vi "Sperre thrust alloc Neptune.vi"(0 "Thruster rpms":dbl[](array[numeric]), 1 "pan tilt":bool[](array[boolean]), 2 "Lights/HMI":bool[](array[boolean]), 5 "error in":errorcluster, 6 "dim 1":i8, 7 "Power Instruments":bool[](array[boolean]), 8 "dim 2":i8, 9 "Collecting Unit":bool[](array[boolean]), 10 "dim 34":i8, 11 "Zoom 1-2":bool[](array[boolean]), 12 "cam no":i8) -> (16 "telebuf out":u8[](array[numeric]), 19 "error IO":errorcluster)   [LabVIEW 2014]
uses:
  <vilib>/imath/engines/lvmath2/RunTimeEngine/BuiltInFunctions/uint8/NIMS_uint8(int).vi
  <instcachedir>/0/NIMS_uint8(int)_9D6EF81F86254677BB00410F9E5C6A1D.lvgen/NIMS_uint8(int)_9D6EF81F86254677BB00410F9E5C6A1D_001.vi
  <vilib>/imath/engines/lvmath2/RunTimeEngine/BuiltInFunctions/round/NIMS_round(DBL-S).vi
  <vilib>/imath/engines/lvmath2/RunTimeEngine/BuiltInFunctions/uint8/NIMS_uint8(real).vi
  <instcachedir>/0/NIMS_uint8(real)_CAA419FBB1354DA296C59E18C46DECF0.lvgen/NIMS_uint8(real)_CAA419FBB1354DA296C59E18C46DECF0_000.vi
  <instcachedir>/0/NIMS_uint8(int)_9D6EF81F86254677BB00410F9E5C6A1D.lvgen/NIMS_uint8(int)_9D6EF81F86254677BB00410F9E5C6A1D_000.vi
  <vilib>/imath/engines/lvmath2/RunTimeEngine/IndexReplace/NIMS V(S)=S.vi
  <instcachedir>/0/NIMS V(S)=S_2D52C4EC15D8415E870AEE69FB516CCA.lvgen/NIMS V(S)=S_2D52C4EC15D8415E870AEE69FB516CCA_003.vi
  <vilib>/imathl/engines/lvmath/Functions/Error Handling/Create Error.vi
  <vilib>/imath/engines/lvmath2/RunTimeEngine/BuiltInFunctions/bitand/NIMS_bitand(SorS,SorS).vi
  <instcachedir>/0/NIMS V(S)=S_2D52C4EC15D8415E870AEE69FB516CCA.lvgen/NIMS V(S)=S_2D52C4EC15D8415E870AEE69FB516CCA_000.vi
  <vilib>/imath/engines/lvmath2/RunTimeEngine/ErrorHandling/NIMS_Create Error From Enums.vi
  <vilib>/imath/engines/lvmath2/RunTimeEngine/IndexRead/NIMS V(S).vi
  <instcachedir>/0/NIMS V(S)_0488751826AF41519A22953C041130DC.lvgen/NIMS V(S)_0488751826AF41519A22953C041130DC_000.vi
  <vilib>/imath/engines/lvmath2/RunTimeEngine/BuiltInFunctions/bitset/NIMS_bitset(RS,RS,RS).vi
  <vilib>/imath/engines/lvmath2/RunTimeEngine/BuiltInFunctions/bitget/NIMS_bitget(SorS,SorS).vi
  <vilib>/imath/engines/lvmath2/RunTimeEngine/RangeToken/NIMS_Range_R2 - Integer.vi
  <instcachedir>/0/NIMS_Range_R2 - Integer_2D1304BAF97744E0A293025746CBADFC.lvgen/NIMS_Range_R2 - Integer_2D1304BAF97744E0A293025746CBADFC_000.vi
  <vilib>/imath/engines/lvmath2/RunTimeEngine/CommandStatement/MC_CommandStatement_break.vi
  <vilib>/imath/engines/lvmath2/RunTimeEngine/BuiltInFunctions/double/NIMS_double.vi
  <instcachedir>/0/NIMS_double_34E32F64C2B04A25A042F4CA881A0A41.lvgen/NIMS_double_34E32F64C2B04A25A042F4CA881A0A41_002.vi
  <vilib>/imath/engines/lvmath2/RunTimeEngine/BuiltInFunctions/mod/NIMS_mod_no_size_check.vi
  <instcachedir>/0/NIMS_mod_no_size_check_5393E3382FD241D281EEB71DA286C65B.lvgen/NIMS_mod_no_size_check_5393E3382FD241D281EEB71DA286C65B_001.vi
  <vilib>/imath/engines/lvmath2/RunTimeEngine/NodeEndStatement/NIMS_NodeEndStatement_Output.vi
  <instcachedir>/0/NIMS_NodeEndStatement_Output_53EC0D466D134D7ABD903AC30B43404B.lvgen/NIMS_NodeEndStatement_Output_53EC0D466D134D7ABD903AC30B43404B_011.vi
  <vilib>/imath/engines/lvmath2/RunTimeEngine/ErrorHandling/NIMS_Finalize Error.vi
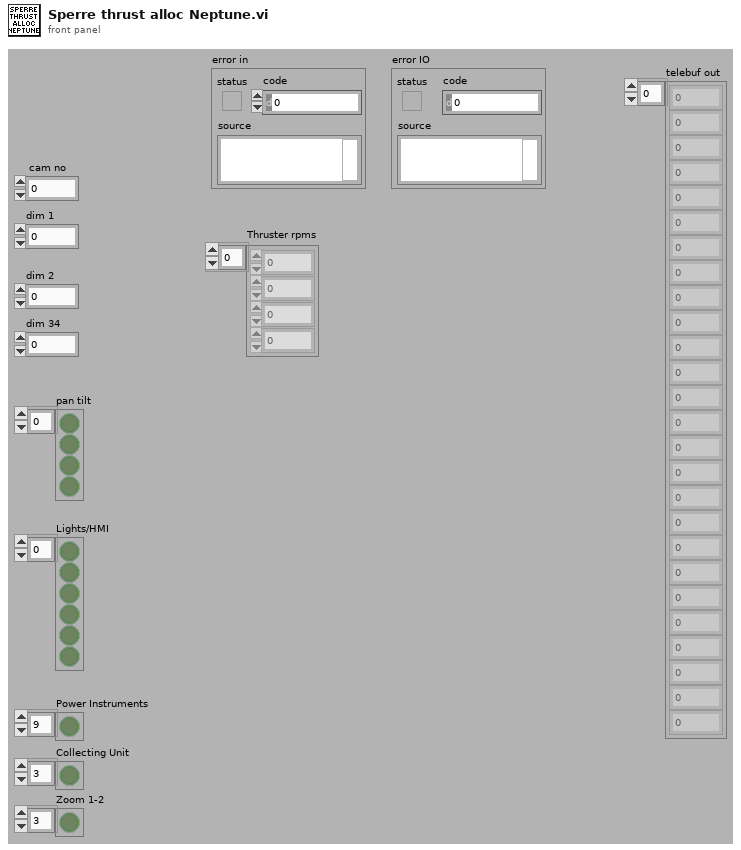
[diagram p1: front panel]
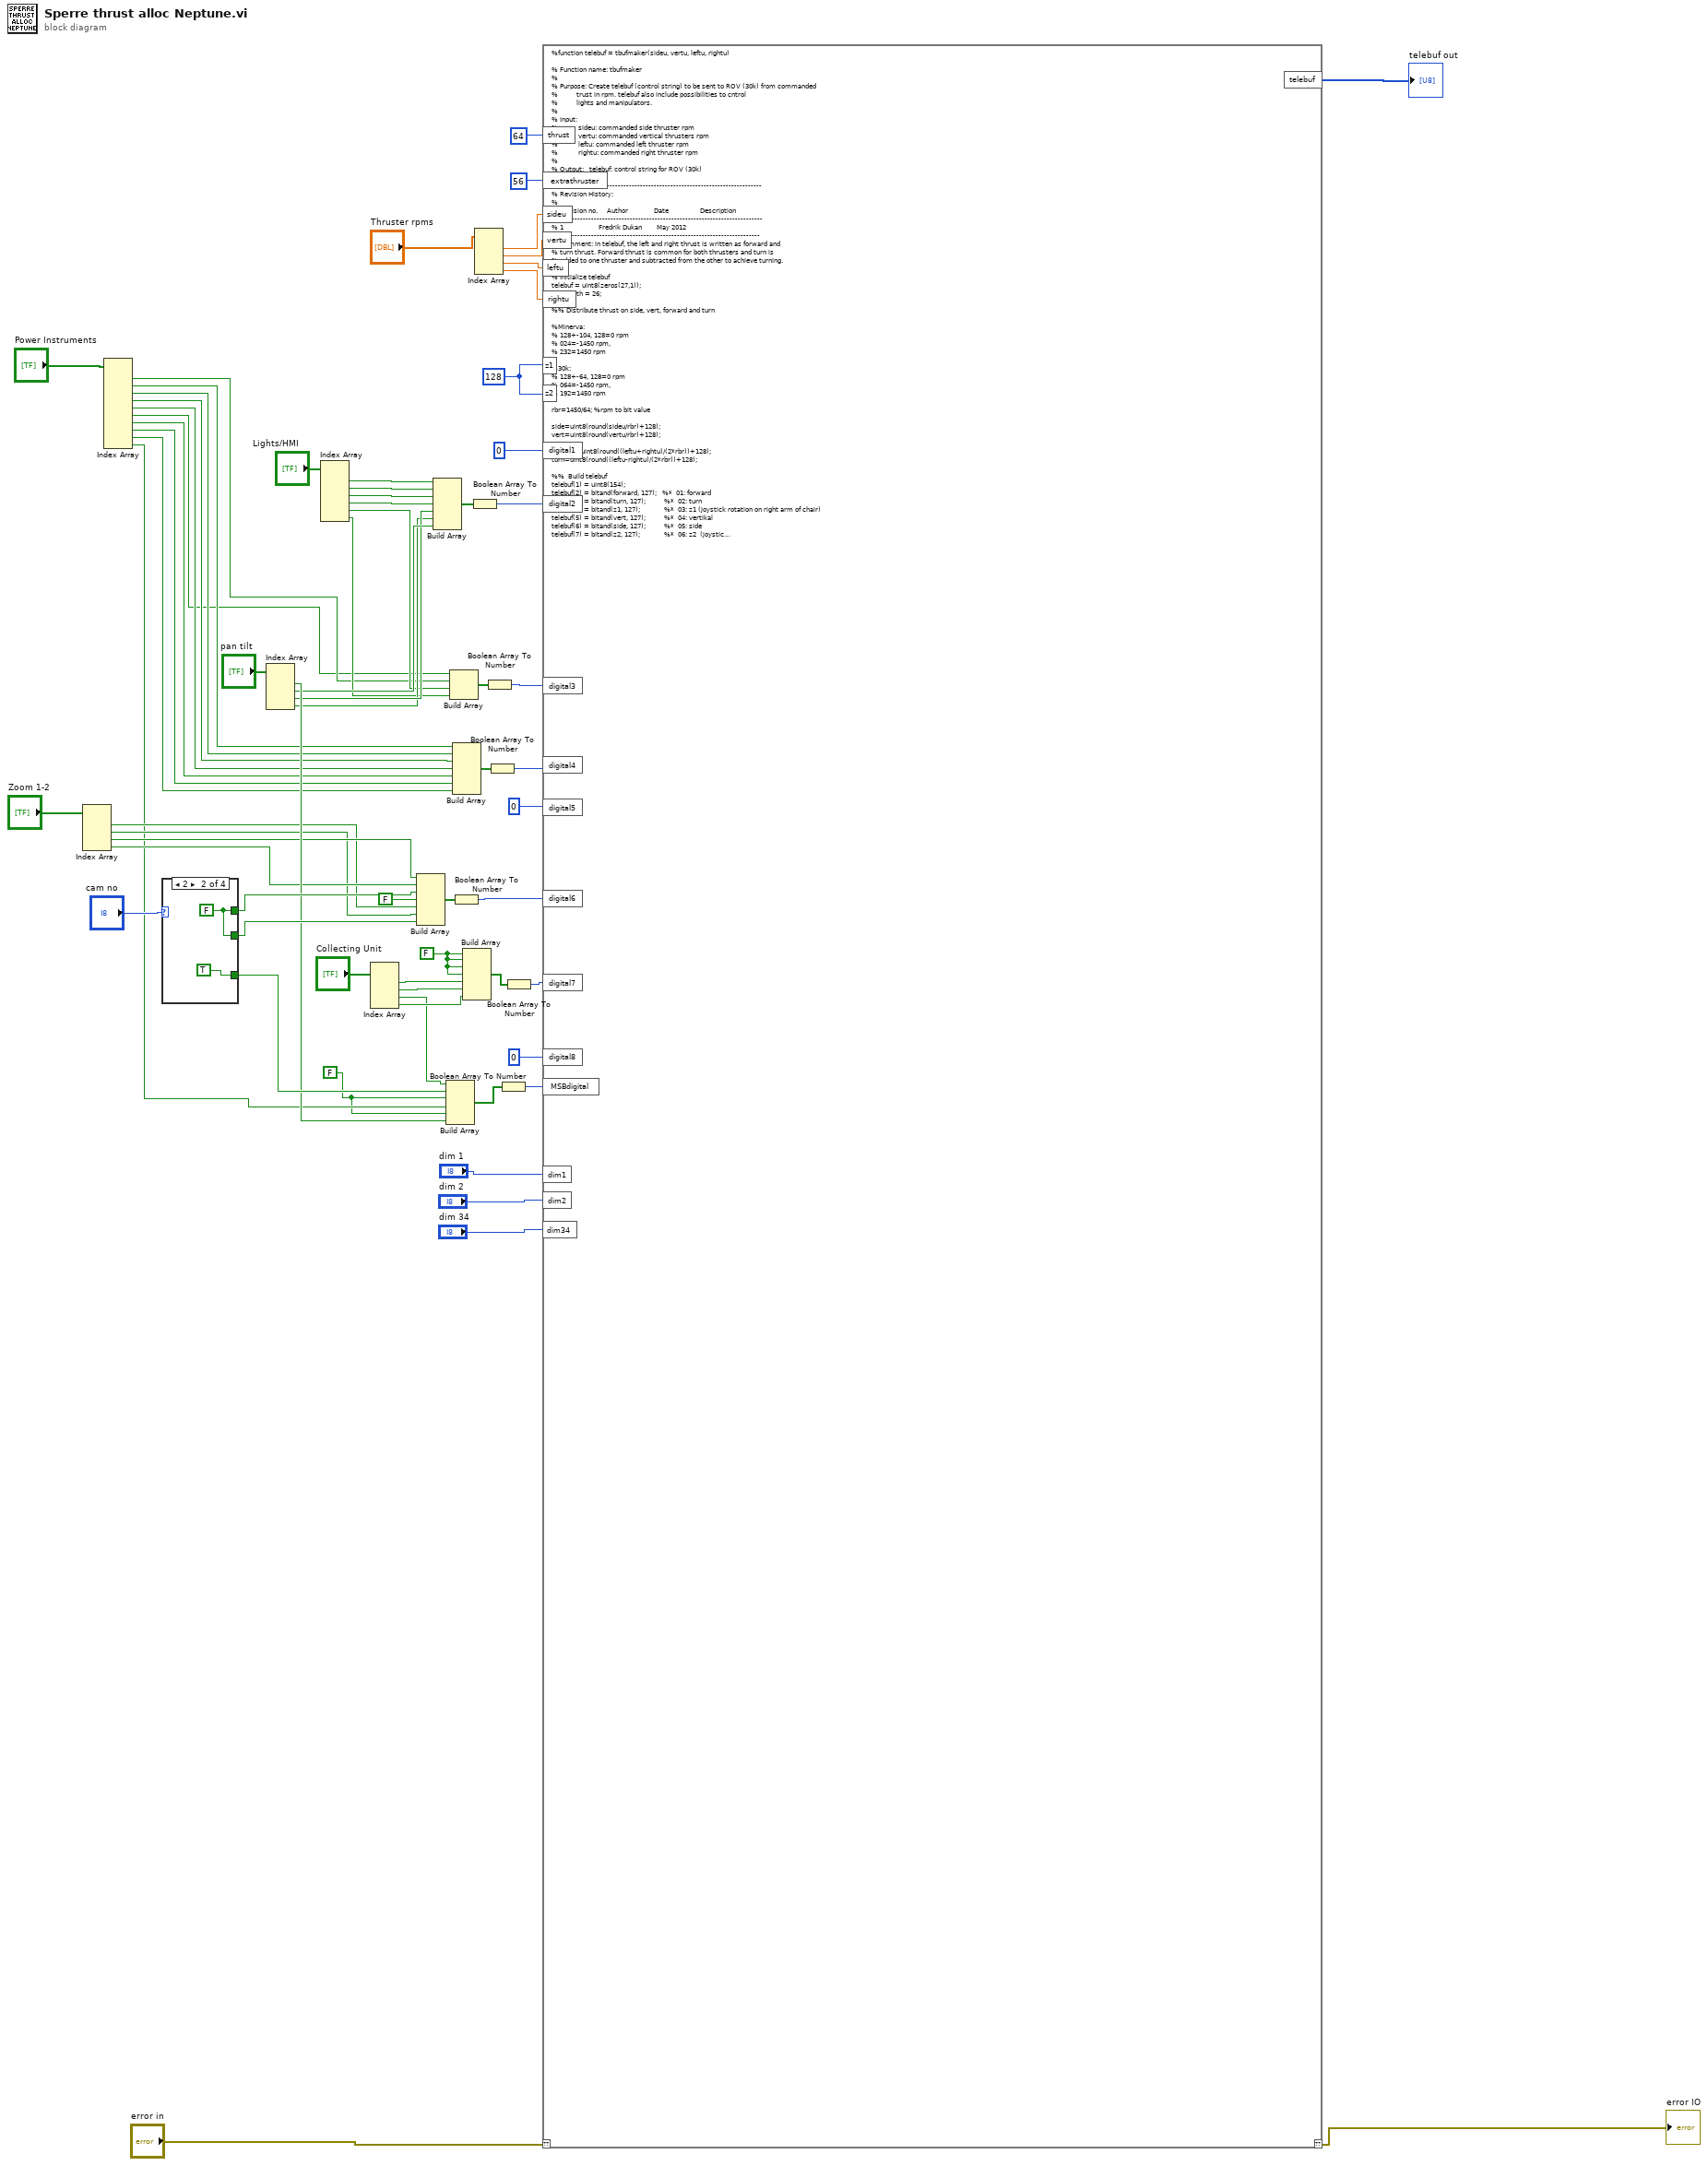
[diagram p0: block diagram]
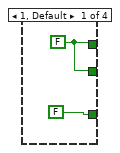
[diagram p2: hidden frame]
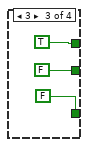
[diagram p3: hidden frame]
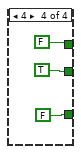
[diagram p4: hidden frame]
diagram:
  w1 = FALSE
  w2 = u8 128 ("digital1")
  w4 = FALSE ("element")
  n1 = Index Array(array="Zoom 1-2") -> (element #1=w8:bool, element #2=w7:bool, element #3=w10:bool, element #4=w9:bool)  [unwired: 4 in]
  n2 = Index Array(array="Power Instruments") -> (element #1=w29:bool, element #2=w24:bool, element #3=w23:bool, element #4=w22:bool, element #5=w21:bool, element #6=w20:bool, element #7=w19:bool, element #8=w18:bool, element #9=w17:bool, element #10=w5:bool)  [unwired: 10 in]
  n3 = case shown="2" "cam no" {
    tunnel: [FALSE ("element") TRUE ("element") FALSE ("element") FALSE ("element")] -> w49
    tunnel: [w70 w72 TRUE ("element") FALSE ("element")] -> w48
    tunnel: [w70 w72 FALSE ("element") TRUE ("element")] -> w47
    frame 1, Default {
      w70 = FALSE ("element")
    }
    frame 2 {
      w72 = FALSE ("element")
    }
    frame 3 {
    }
    frame 4 {
    }
  }
  n4 = Index Array(array="pan tilt") -> (element #1=w43:bool, element #2=w42:bool, element #3=w41:bool, element #4=w40:bool)  [unwired: 4 in]
  n5 = Index Array(array="Lights/HMI") -> (element #1=w38:bool, element #2=w37:bool, element #3=w36:bool, element #4=w35:bool, element #5=w34:bool, element #6=w33:bool)  [unwired: 6 in]
  n6 = Index Array(array="Collecting Unit") -> (element #1=w14:bool, element #2=w13:bool, element #3=w11:bool, element #4=w12:bool)  [unwired: 4 in]
  n7 = Build Array(w10, w9, w48, FALSE ("element"), w8, w7, w47) -> (w53:bool[])
  n8 = Build Array(w38, w37, w36, w35, w41, w40, w42) -> (w67:bool[])
  n9 = Build Array(w11, w49, w4, w5, w4, w43) -> (w51:bool[])
  n10 = Build Array(w20, w29, w34, w33) -> (w57:bool[])
  n11 = Build Array(w24, w23, w22, w21, w19, w18, w17) -> (w26:bool[])
  n12 = Boolean Array To Number(Boolean array=w53) -> (number=w52:u32)
  n13 = Build Array(w1, w1, w1, w1, w14, w13, w12) -> (w16:bool[])
  n14 = Boolean Array To Number(Boolean array=w67) -> (number=w55:u32)
  n15 = Index Array(array="Thruster rpms") -> (element #1=w62:dbl, element #2=w61:dbl, element #3=w60:dbl, element #4=w59:dbl)  [unwired: 4 in]
  n16 = Boolean Array To Number(Boolean array=w57) -> (number=w56:u32)
  n17 = Boolean Array To Number(Boolean array=w26) -> (number=w25:u32)
  n18 = Boolean Array To Number(Boolean array=w51) -> (number=w50:u32)
  n19 = Boolean Array To Number(Boolean array=w16) -> (number=w15:u32)
  n20 = mathscript code="%function telebuf = tbufmaker(sideu, vertu, leftu, rightu)\n\n% Function name: tbufmaker\n%\n% Purpose: Create telebuf (control string) to be sent to ROV (30k) from commanded\n%          trust in rpm. telebuf also include possibilities to cntrol\n%          lights and manipulators.\n%\n% Input:  \n%           sideu: commanded side thruster rpm\n%           vertu: commanded vertical thrusters rpm\n%           leftu: commanded left thruster rpm\n%           rightu: commanded right thruster rpm\n%\n% Output:   telebuf: control string for ROV (30k)\n%\n% -------------------------------------------------------------------------\n% Revision History:\n%\n% Revision no.     Author              Date                 Description\n%--------------------------------------------------------------------------\n% 1                   Fredrik Dukan        May 2012\n%-------------------------------------------------------------------------\n% Comment: in telebuf, the left and right thrust is written as forward and\n% turn thrust. Forward thrust is common for both thrusters and turn is \n% added to one thruster and subtracted from the other to achieve turning.\n\n% Initialize telebuf\ntelebuf = uint8(zeros(27,1));\ntelelength = 26;\n\n%% Distribute thrust on side, vert, forward and turn\n\n%Minerva:\n% 128+-104, 128=0 rpm\n% 024=-1450 rpm,\n% 232=1450 rpm\n\n%30k:\n% 128+-64, 128=0 rpm\n% 064=-1450 rpm,\n% 192=1450 rpm\n\nrbr=1450/64; %rpm to bit value\n\nside=uint8(round(sideu/rbr)+128);\nvert=uint8(round(vertu/rbr)+128);\n\nforward=uint8(round((leftu+rightu)/(2*rbr))+128);\nturn=uint8(round((leftu-rightu)/(2*rbr))+128);\n\n%%  Build telebuf\ntelebuf(1) = uint8(154);\ntelebuf(2) = bitand(forward, 127);   %*  01: forward\ntelebuf(3) = bitand(turn, 127);          %*  02: turn\ntelebuf(4) = bitand(z1, 127);             %*  03: z1 (joystick rotation on right arm of chair)\ntelebuf(5) = bitand(vert, 127);          %*  04: vertikal\ntelebuf(6) = bitand(side, 127);          %*  05: side\ntelebuf(7) = bitand(z2, 127);             %*  06: z2  (joystick rotation on left arm of chair)\n\ntelebuf(8) = bitset(uint8(telebuf(8)), 7, 0); % note: not needed in matlab   %*  07: MSB thruster\ntelebuf(8) = bitset(uint8(telebuf(8)), 7, bitget(forward, 8));\ntelebuf(8) = bitset(uint8(telebuf(8)), 6, 0); % note: not needed in matlab\ntelebuf(8) = bitset(uint8(telebuf(8)), 6, bitget(turn, 8));\ntelebuf(8) = bitset(uint8(telebuf(8)), 5, 0); % note: not needed in matlab\ntelebuf(8) = bitset(uint8(telebuf(8)), 5, bitget(z1, 8)); % note: not needed in matlab\ntelebuf(8) = bitset(uint8(telebuf(8)), 4, 0); % note: not needed in matlab\ntelebuf(8) = bitset(uint8(telebuf(8)), 4, bitget(vert, 8));\ntelebuf(8) = bitset(uint8(telebuf(8)), 3, 0); % note: not needed in matlab\ntelebuf(8) = bitset(uint8(telebuf(8)), 3, bitget(side, 8)); \ntelebuf(8) = bitset(uint8(telebuf(8)), 2, 0); % note: not needed in matlab\ntelebuf(8) = bitset(uint8(telebuf(8)), 2, bitget(z2, 8)); % note: not needed in matlab\n\ntelebuf(9) = thrust;     %*  08: thrust  (vertical thrust knob)\ntelebuf(10) = dim1;     %*  09: dimmer 1\ntelebuf(11) = dim2;     %*  10: dimmer 2\ntelebuf(12) = dim34;   %*  11: dimmer 3+4\n\n%*  12: spare 1\n%*  13: spare 2\n\ntelebuf(15) =uint8(56); %*  14: extra thruster\ntelebuf(16) =digital1;    %*  15: digital 1\ntelebuf(17) =digital2;    %*  16: digital 2\ntelebuf(18) =digital3;    %*  17: digital 3\ntelebuf(19) =digital4;    %*  18: digital 4\ntelebuf(20) =digital5;     %*  19: digital 5\ntelebuf(21) =digital6;     %*  20: digital 6\ntelebuf(22) =digital7;     %*  21: digital 7\ntelebuf(23) =digital8;     %*  22: digital 8\n\ntelebuf(24) =MSBdigital;   %*  23: MSB digital\n%checksums\n%telebuf(13) = bitand(uint8(telebuf(13)), uint8(59)); %turn off auto heading and depth   \n\nchk = uint8(0);\n\nfor i = 1:telelength - 1\n    chk = chk + telebuf(i);\nend\nchk1 = double(chk);\ncheck1 = bitand(uint8(floor(chk1/256)), 127);\ncheck2 = bitand(mod(chk, 256) , 127);\ntelebuf(26) = check1;   %*  25: checksum 1\ntelebuf(27) = check2;   %*  26: checksum 2\n\n%\n%/* Dataformat:\n% RS232\n%* 9600,n,8,1\n%*/\n \n%/*\n%*  the receive-data-from-surface process\n%*\n%*  data are received on the B-port of QUART\n%*\n%*  telegram format (26 bytes) :\n%*  7 bits for data, bit 8 (0x80(hex80)) is startbit.\n \n %*  00: start  (0x9C)  (startbit + telegram length)\n%*  01: forward\n%*  02: turn\n%*  03: z1\n%*  04: vertikal\n%*  05: side\n%*  06: z2\n%*  07: MSB thruster\n%*  08: thrust\n%*  09: dimmer 1\n%*  10: dimmer 2\n%*  11: dimmer 3+4\n%*  12: spare 1\n%*  13: spare 2\n%*  14: extra thruster\n%*  15: digital 1\n%*  16: digital 2\n%*  17: digital 3\n%*  18: digital 4\n%*  19: digital 5\n%*  20: digital 6\n%*  21: digital 7\n%*  22: digital 8\n%*  23: MSB digital\n%*  24: AF digital\n%*  25: checksum 1\n%*  26: checksum 2"("??"="error in", "sideu"=w62, "vertu"=w61, "leftu"=w60, "rightu"=w59, "dim1"="dim 1", "dim2"="dim 2", "digital1"=i8 0, "digital2"=w55, "digital3"=w56, "dim34"="dim 34", "digital6"=w52, "MSBdigital"=w50, "thrust"=i8 64 ("digital1"), "extrathruster"=i8 56 ("digital1"), "digital4"=w25, "digital5"=i8 0 ("digital1"), "digital7"=w15, "digital8"=i8 0 ("digital1"), "z1"=w2, "z2"=w2) -> ("??"=→"error IO":errorcluster, "telebuf"=→"telebuf out":u8[])
